vi "StartDetectorControlVI.vi"(8 "entrée d'erreur (pas d'erreur)":errorcluster, 11 "Control en entrée":refnum<class "Control-Server.lvclass">) -> (0 "sortie d'erreur":errorcluster, 3 "Control en sortie":refnum<class "Control-Server.lvclass">)   [LabVIEW 2015, in "Control-Server.lvclass"]
uses:
  Classes/Control/Control-Server/Control-Server.lvclass
  Classes/Control/Control-Server/Control-Server.lvclass/Control-Server.ctl
  Clusters-def/Message types.ctl
  Classes/Message/Message.lvclass/Message.ctl
  Classes/Detector/Detector.lvclass
  Classes/Message/Message.lvclass
  Classes/GeneralFunctionality/GeneralFunctionality.lvclass
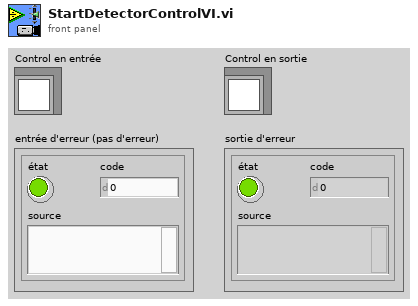
[diagram p1: front panel]
types:
  T1 = typedef "Message types.ctl" = string
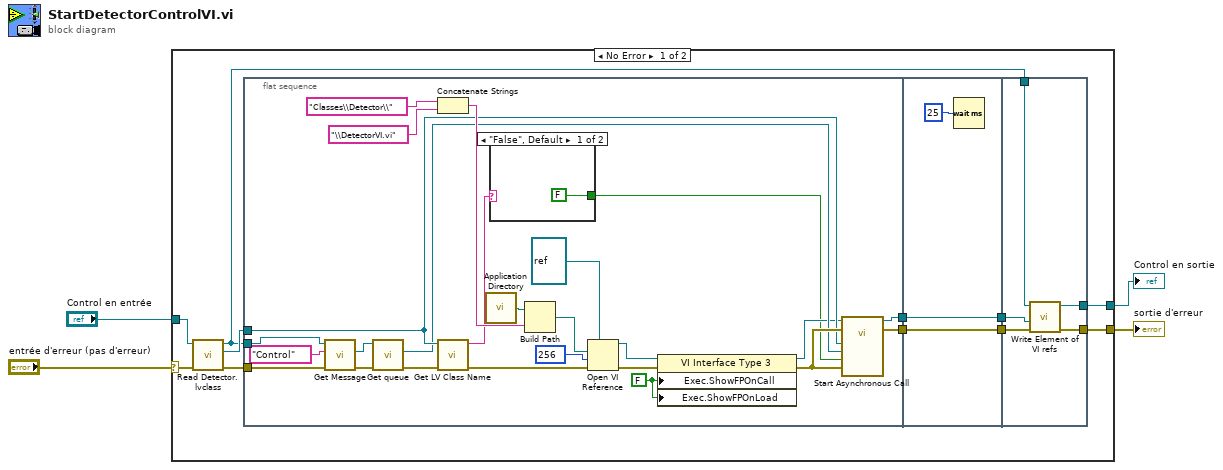
[diagram p0: block diagram]
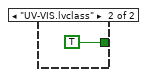
[diagram p2: hidden frame]
diagram:
  n1 = case shown="No Error" "entrée d'erreur (pas d'erreur)" {
    selector: "entrée d'erreur (pas d'erreur)" -> [w12 w52]
    tunnel: [w9 w51] -> w4
    tunnel: [w10 w52] -> w3
    tunnel: "Control en entrée" -> [w13 w51]
    frame No Error {
      n2 = call "Read Detector.lvclass.vi"("error in (no error)"=w12, "Control in"=w13) -> ("error out"=w14:errorcluster, "Detector.lvclass"=w15:refnum<class "Detector.lvclass">, "Control out"=w11:refnum<class "Control-Server.lvclass">)  [unwired: 7 in]
      n3 = flat-sequence {
        tunnel: w15 -> [w21]
        tunnel: w14 -> [w26]
        tunnel: [w40] -> w8
        tunnel: [w27] -> w6
        tunnel: w11 -> [w25]
        tunnel: w8 -> [w45]
        tunnel: [w45] -> w7
        tunnel: w6 -> [w44]
        tunnel: [w44] -> w5
        tunnel: w7 -> [w47]
        tunnel: w5 -> [w50]
        tunnel: w11 -> [w46]
        tunnel: [w48] -> w10
        tunnel: [w49] -> w9
        frame #0 {
          w29 = FALSE ("Exécution:Afficher la face-avant à l'appel")
          n4 = call "Get Message.vi"("error in (no error)"=w26, "Message type"=T1 "Control", "GeneralFunctionality en entrée"=w25) -> ("error out"=w22:errorcluster, "Message.lvclass"=w23:refnum<class "Message.lvclass">)  [unwired: 6 in, 1 out]
          n5 = call "Get queue.vi"("error in (no error)"=w22, "Message in"=w23) -> ("error out"=w19:errorcluster, "queue"=w20:refnum<queue>)  [unwired: 7 in, 1 out]
          n6 = Concatenate Strings("Classes\\Detector\\" ("chaîne"), "\\DetectorVI.vi" ("chaîne")) -> (w37:string)
          n7 = call <vilib>:"Get LV Class Name.vi"("error in (no error)"=w19, "object"=w21) -> ("error out"=w33:errorcluster, "class name"=w17:string)  [unwired: 8 in]
          n8 = call <vilib>:"Application Directory.vi"() -> ("Application Directory"=w35:path)
          n9 = case shown="\"False\", Default" w17 {
            tunnel: [FALSE TRUE] -> w16
            frame "False", Default {
            }
            frame "UV-VIS.lvclass" {
            }
          }
          n10 = Build Path(base path=w35, name or relative path=w37) -> (appended path=w34:path)
          n11 = Open VI Reference(type specifier VI Refnum (for type only)=refnum<vi> refnum ("spécificateur de type du refnum de VI (pour type seulement)"), vi path=w34, options=256, error in (no error)=w33) -> (vi reference=w31:refnum<vi>, error out=w30:errorcluster)  [unwired: 2 in]
          n12 = property class="VI Interface Type 3"(reference=w31, error in=w30, "Exec.ShowFPOnCall"=w29, "Exec.ShowFPOnLoad"=w29) -> (reference out=w18:refnum<vi>, error out=w32:errorcluster)
          n13 = call-by-ref "Start Asynchronous Call"(reference=w18, error in=w32, 8:"error in (no error)"=w32, "Visible"=w16, "ControlQueue"=w20, "Detector.lvclass"=w21) -> (reference out=w27:refnum<vi>, error out=w40:errorcluster)  [unwired: 7 in, 1 out]
        }
        frame #1 {
          n14 = Wait (ms)(milliseconds to wait=u32 25) -> ()  [unwired: 1 out]
        }
        frame #2 {
          n15 = call "Write Element of VI refs.vi"("error in (no error)"=w47, "vi reference"=w50, "Control in"=w46) -> ("error out"=w48:errorcluster, "Control out"=w49:refnum<class "Control-Server.lvclass">)  [unwired: 7 in]
        }
      }
    }
    frame Error {
    }
  }
  "Control en sortie" <- w4
  "sortie d'erreur" <- w3
